vi "Comparador_de_nivel.vi"(10 "Numeric":dbl, 11 "Numeric in":dbl) -> (3 "Numeric 2":i16)   [LabVIEW 2016]
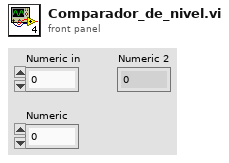
[diagram p1: front panel]
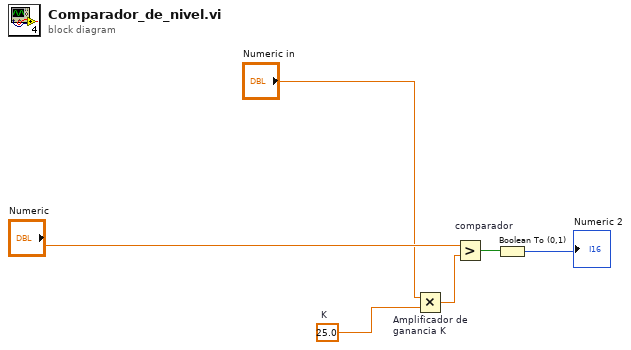
[diagram p0: block diagram]
diagram:
  w5 = 25.0  # K
  n1 = Multiply "Amplificador de ganancia K"(x="Numeric in", y=w5) -> (x*y=w1:dbl)
  n2 = Greater? "comparador"(x="Numeric", y=w1) -> (0:w3:bool)
  n3 = Boolean To (0,1)(Boolean=w3) -> (0, 1=→"Numeric 2":i16)
